vi "24HP test panel - USB - external control.vi"(2 "Datalog file path (full)":path, 3 "COM port":refnum<visa-resource-name>, 4 "Log data stream":bool, 5 "Data rate (Hz)":u8(ring)=14 items=["1", "2", "4", "5", "8", "10", "16", "20", "25", "32", "40", "50", "64", "80", "100", "125", "160", "200", "250", "320", "400", "500", "625", "800", "1000"], 6 "N samples":u32=1000, 7 "Command":T2="D") -> (0 "Error":errorcluster, 1 "Data out":T3[](array[typedef]) {"Time stamp" format="%<%.6X\n%x>T"})   [LabVIEW 2020]
uses:
  ctls/24HP_Cmd (USB).ctl
  ctls/24HP_Data cluster.ctl
  Globals/Meas_global.vi
panel:
  in  "Main":T1(tab)
  out "Serial number":u32
  out "Subsystems ok":bool[](array[boolean])
  out "Pressure sensor values in range":bool[](array[boolean])
  out "Pressure sensor status good":bool[](array[boolean])
  out "P_offset_table_auto_zero":sgl[][](array[numeric]) format="%#_6f"
  out "n":u16
  out "Auto zero progBar":u16(slide) caption="Collecting samples, please maintain dP = 0" scale=0.0..100.0
  in  "P_atm offset (Pa)":sgl
  in  "T_external offset (°C)":sgl
  in  "Data period on power-up (ms)":u32=10000
  in  "TTL baud rate (bps)":u32=500000
  in  "Serial number":u32=9999
  in  "IMU params 2":u8[](array[numeric])=[0, 0, 4]
  in  "IMU params 1":sgl[](array[numeric])=[1.0, 0.0, 0.0, 0.0]
  in  "P_offset_table":sgl[][](array[numeric])=[[0.0, 0.0, 0.0, 0.0, 0.0, 0.0, 0.0, 0.0], [0.0, 0.0, 0.0, 0.0, 0.0, 0.0, 0.0, 0.0], [0.0, 0.0, 0.0, 0.0, 0.0, 0.0, 0.0, 0.0]] format="%#_6f"
  in  "Power-up defaults":u8[](array[numeric])=[0, 3, 0, 0]
  out "Chk ok":bool
  out "EEPROM Checksum":u16 format="%04x"
  out "received":bool
  out "Returned data rate (Hz)":u32
  out "sent":bool
  out "w_xyz (dps)":sgl[](array[numeric])
  out "a_xyz (g)":sgl[](array[numeric])
  out "T_external (°C)":sgl format="%#_4f"
  out "T_board (°C)":sgl format="%#_4f"
  out "Sensor status":bool[][][](array[boolean])
  out "frm err":u32
  out "chk err":u32
  in  "Stop Data":bool
  out "Checksum ok":bool
  out "Stream enabled":bool
  out "Pressures":sgl[][](graph)
  out "Rel. hum (%)":sgl format="%#_4f"
  out "P_atm (mbar)":sgl format="%#_4f"
  # "Paul Nathan"
  # "11/2021"
  # "On-board temperature sensor ok"
  # "External temperature sensor ok"
  # "MCU EEPROM checksum ok"
  # "IMU detected"
  # "Accelerometer self test pass"
  # "Gyroscope self test pass"
  # "Env. sensor detected"
  # "Bank 0 pressure sensor values in range"
  # "Bank 1 pressure sensor values in range"
  # "Bank 2 pressure sensor values in range"
  # "Bank 0 pressure sensor statuses good"
  # "Bank 1 pressure sensor statuses good"
  # "Bank 2 pressure sensor statuses good"
  # "%"
  # "P0 offset"
  # "P1 offset"
  # "P2 offset"
  # "P3 offset"
  # "P4 offset"
  # "P5 offset"
  # "P6 offset"
  # "P7 offset"
  # "Bank 2"
  # "Bank 1"
  # "Bank 0"
  # "acc range mode"
  # "gyr range mode"
  # "IMU update rate mode"
  # "a_xyz scale"
  # "w_x offset (dps)"
  # "w_y offset (dps)"
  # "w_z offset (dps)"
  # "P0 offset"
  # "P1 offset"
  # "P2 offset"
  # "P3 offset"
  # "P4 offset"
  # "P5 offset"
  # "P6 offset"
  # "P7 offset"
  # "Bank 2"
  # "Bank 1"
  # "Bank 0"
  # "TTL data output on power-up"
  # "Number of active sensor banks"
  # "Sleep sensors after data stream"
  # "Sync sensor and data clocks"
  # "bank"
  # "0"
  # "1"
  # "2"
  # "3"
  # "4"
  # "5"
  # "6"
  # "7"
  # "Powered"
  # "!Busy"
  # "!MemErr"
  # "!MathSat"
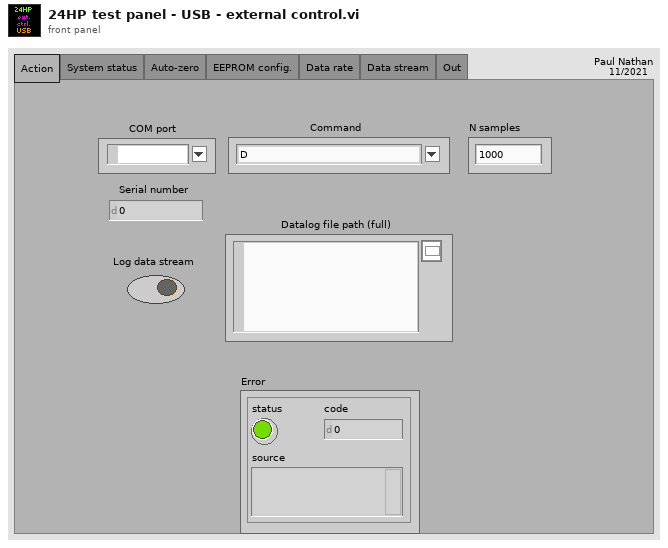
[diagram p1: front panel]
types:
  T1 = enum32{"Action", "System status", "Auto-zero", "EEPROM config.", "Data rate", "Data stream", "Out"}
  T2 = typedef "24HP_Cmd (USB).ctl" = string
  T3 = typedef "24HP_Data cluster.ctl" = cluster{"Time stamp":timestamp, "Pressures (Pa)":sgl[], "T_external (°C)":sgl, "T_board (°C)":sgl, "P_atm (mbar)":sgl, "Rel. hum. (%)":sgl, "a_xyz (g)":sgl[], "w_xyz (dps)":sgl[], "Status bytes":u8[]}
  T4 = enum32{"Action", "System status", "Auto-zero", "EEPROM config.", "Data rate", "Data stream"}
  T5 = enum16{"open", "replace", "create", "open or create", "replace or create", "replace or create with confirmation"}
  T6 = typedef "Rendezvous RefNum" = refnum<k1>
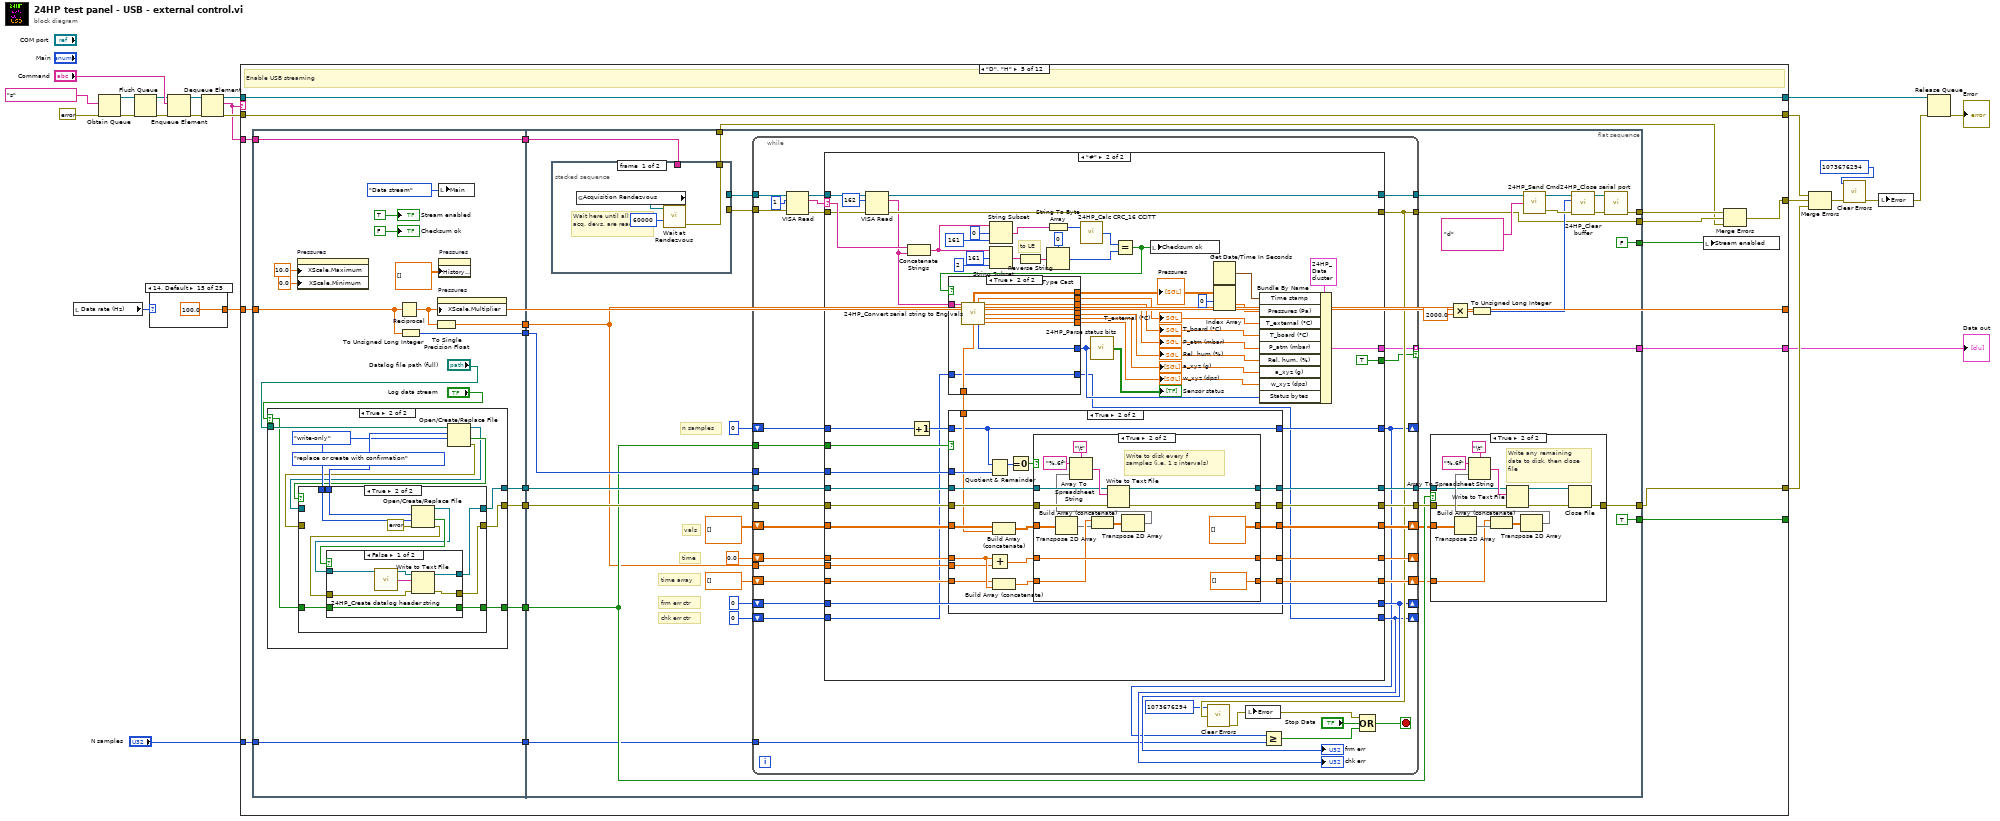
[diagram p0: block diagram]
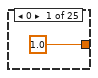
[diagram p2: hidden frame]
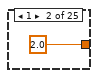
[diagram p3: hidden frame]
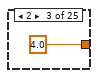
[diagram p4: hidden frame]
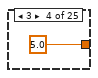
[diagram p5: hidden frame]
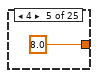
[diagram p6: hidden frame]
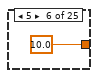
[diagram p7: hidden frame]
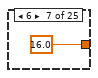
[diagram p8: hidden frame]
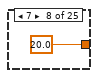
[diagram p9: hidden frame]
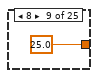
[diagram p10: hidden frame]
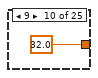
[diagram p11: hidden frame]
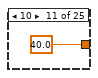
[diagram p12: hidden frame]
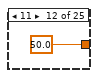
[diagram p13: hidden frame]
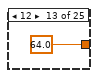
[diagram p14: hidden frame]
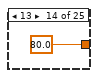
[diagram p15: hidden frame]
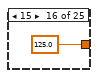
[diagram p16: hidden frame]
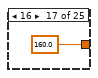
[diagram p17: hidden frame]
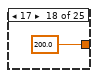
[diagram p18: hidden frame]
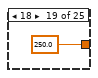
[diagram p19: hidden frame]
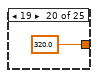
[diagram p20: hidden frame]
diagram:
  n1 = local read "Data rate (Hz)"() -> (w6:u8)
  n2 = Obtain Queue(element data type=T2 "s" ("Combo Box"), error in (no error)=errorcluster {"status"=FALSE, "code"=0, "source"=""}) -> (queue out=w22:refnum<queue>, error out=w23:errorcluster)  [unwired: 3 in, 1 out]
  n3 = Flush Queue(queue=w22, error in (no error)=w23) -> (queue out=w16:refnum<queue>, error out=w15:errorcluster)  [unwired: 1 out]
  n4 = case shown="14, Default" w6 {
    tunnel: [1.0 2.0 4.0 5.0 8.0 10.0 16.0 20.0 25.0 32.0 40.0 50.0 64.0 80.0 100.0 125.0 160.0 200.0 250.0 320.0 400.0 500.0 625.0 800.0 1000.0] -> w5
    frame 0 {
    }
    frame 1 {
    }
    frame 2 {
    }
    frame 3 {
    }
    frame 4 {
    }
    frame 5 {
    }
    frame 6 {
    }
    frame 7 {
    }
    frame 8 {
    }
    frame 9 {
    }
    frame 10 {
    }
    frame 11 {
    }
    frame 12 {
    }
    frame 13 {
    }
    frame 14, Default {
    }
    frame 15 {
    }
    frame 16 {
    }
    frame 17 {
    }
    frame 18 {
    }
    frame 19 {
    }
    frame 20 {
    }
    frame 21 {
    }
    frame 22 {
    }
    frame 23 {
    }
    frame 24 {
    }
  }
  n5 = Enqueue Element(queue=w16, element="Command", error in (no error)=w15) -> (queue out=w20:refnum<queue>, error out=w19:errorcluster)  [unwired: 1 in, 1 out]
  n6 = Dequeue Element(queue=w20, error in (no error)=w19) -> (queue out=w14:refnum<queue>, element=w12:T2, error out=w13:errorcluster)  [unwired: 1 in, 1 out]
  n7 = case shown="\"D\", \"H\"" w12 {
    tunnel: [w56 w93 w144 w269 w378 w664 w691 w753 w795 w824 FALSE FALSE] -> _
    tunnel: w14 -> [w55 w92 w143 w272 w377 w666 w693 w755 w794 w816 w840 w845]
    tunnel: [w55 w92 w143 w272 w377 w666 w693 w755 w794 w815 w840 w845] -> w4
    tunnel: w13 -> [w54 w91 w142 w271 w376 w665 w694 w756 w793 w823 w839 w844]
    tunnel: [w54 w91 w142 w271 w376 w665 w694 w756 w793 w823 w839 w844] -> w11
    tunnel: w12 -> [w53 w90 w141 w277 w375 w668 w698 w761 w792 w822 _ _]
    tunnel: [w51 w88 w139 w270 w363 w667 w692 w754 w790 w817 errorcluster {"status"=FALSE, "code"=0, "source"=""} ("Error out") errorcluster {"status"=FALSE, "code"=0, "source"=""} ("Error out")] -> w10
    tunnel: [_ _ _ _ w373 _ _ _ _ _ _ _] -> w9
    tunnel: w5 -> [w50 w87 w138 w274 w366 w662 _ _ w789 w820 w836 w841]
    tunnel: [w50 w87 w138 w274 w366 w662 w690 w757 w789 w820 w836 w841] -> _
    tunnel: [_ _ _ _ w362 _ _ _ _ _ _ _] -> w2
    tunnel: "N samples" -> [_ _ _ _ w361 _ _ _ _ _ _ _]
    frame "S", "s" {
      # "Perform self-test and retrieve status bytes, Retrieve status bytes"
      n8 = flat-sequence {
        tunnel: w53 -> [w59]
        tunnel: [w59] -> w52
        tunnel: [TRUE] -> w56
        tunnel: w52 -> [w64]
        tunnel: [w63] -> w51
        frame #0 {
          w58 = bool[] [] ("Pressure sensor EEPROM checksums ok")
          n9 = local write "Main"(T4."System status" ("Main")) -> ()
          "Pressure sensor status good" <- w58
          "Pressure sensor values in range" <- w58
          "Subsystems ok" <- w58
        }
        frame #1 {
          w68 = 1 ("length (rest)")
          w75 = u8 0 ("byte count")
          n10 = local read "COM port"() -> (w65:refnum<visa-resource-name>)
          n11 = call "24HP_Open serial port.vi"("timeout (ms)"=u32 5000, "VISA resource name"=w65) -> ("Error out"=w84:errorcluster, "VISA resource name out"=w85:refnum<visa-resource-name>)  [unwired: 8 in]
          n12 = call "24HP_Send Cmd.vi"("Error In"=w84, "Operation"=w64, "Port"=w85) -> ("Error Out"=w82:errorcluster, "Port out"=w83:refnum<visa-resource-name>)  [unwired: 1 in]
          n13 = VISA Read(VISA resource name=w83, byte count=u32 3, error in (no error)=w82) -> (VISA resource name out=w80:refnum<visa-resource-name>, read buffer=w71:string, error out=w79:errorcluster)  [unwired: 1 out]
          n14 = call "24HP_Close serial port.vi"("Error in"=w79, "VISA resource name"=w80) -> ("Error out"=w63:errorcluster)  [unwired: 9 in]
          n15 = String Subset(string=w71, offset (0)=0, length (rest)=w68) -> (substring=w78:string)
          n16 = String Subset(string=w71, offset (0)=1, length (rest)=w68) -> (substring=w77:string)
          n17 = String Subset(string=w71, offset (0)=2 ("length (rest)"), length (rest)=w68) -> (substring=w76:string)
          n18 = Type Cast(type=w75, x=w78) -> (*(type *) &x=w74:u8)
          n19 = Type Cast(type=w75, x=w77) -> (*(type *) &x=w73:u8)
          n20 = Type Cast(type=w75, x=w76) -> (*(type *) &x=w72:u8)
          n21 = Number To Boolean Array(number=w74) -> (Boolean array=w62:bool[])
          n22 = Number To Boolean Array(number=w73) -> (Boolean array=w61:bool[])
          n23 = Number To Boolean Array(number=w72) -> (Boolean array=w60:bool[])
          n24 = local write "Pressure sensor values in range"(w62) -> ()
          n25 = local write "Pressure sensor status good"(w61) -> ()
          n26 = local write "Subsystems ok"(w60) -> ()
        }
      }
    }
    frame "Z", "z" {
      # "Perform permanent auto-zero (write values to EEPROM), Perform temporary auto-zero"
      n27 = flat-sequence {
        tunnel: w90 -> [w97]
        tunnel: [w97] -> w89
        tunnel: [TRUE] -> w93
        tunnel: w89 -> [w109]
        tunnel: [w106] -> w88
        frame #0 {
          n28 = local write "Main"(T4."Auto-zero" ("Main")) -> ()
          "P_offset_table_auto_zero" <- sgl[][] [] ("P_raw_Azero")
          "Auto zero progBar" <- u16 0 ("Collecting samples, please maintain dP = 0")
        }
        frame #1 {
          w98 = 3  # N banks
          # "Reverse columns to match physical layout"
          n29 = local read "COM port"() -> (w110:refnum<visa-resource-name>)
          n30 = call "24HP_Open serial port.vi"("timeout (ms)"=u32 16000, "VISA resource name"=w110) -> ("Error out"=w117:errorcluster, "VISA resource name out"=w118:refnum<visa-resource-name>)  [unwired: 8 in]
          n31 = call "24HP_Send Cmd.vi"("Error In"=w117, "Operation"=w109, "Port"=w118) -> ("Error Out"=w115:errorcluster, "Port out"=w116:refnum<visa-resource-name>)  [unwired: 1 in]
          n32 = VISA Read(VISA resource name=w116, byte count=u32 96, error in (no error)=w115) -> (VISA resource name out=w113:refnum<visa-resource-name>, read buffer=w107:string, error out=w112:errorcluster)  [unwired: 1 out]
          n33 = for {
            N: 100 -> [_]
            shift-right: [w127] -> _
            shift-left: u16 0 -> [w128]
            n34 = Increment(x=w128) -> (x+1=w127:u16)
            "n" <- w127
            n35 = Wait (ms)(milliseconds to wait=u32 100) -> ()  [unwired: 1 out]
            n36 = local write "Auto zero progBar"(w127) -> ()
          }
          n37 = for {
            N: 24 -> [_]
            tunnel: [w131] -> w99 mode=indexing
            tunnel: w107 -> [w130]
            i -> [w137]
            w135 = 4 ("x")
            # "to BE"
            n38 = Multiply(x=w135, y=w137) -> (x*y=w136:i32)
            n39 = String Subset(string=w130, offset (0)=w136, length (rest)=w135) -> (substring=w134:string)
            n40 = Reverse String(1:w134) -> (0:w133:string)
            n41 = Type Cast(type=sgl 0.0 ("byte count"), x=w133) -> (*(type *) &x=w131:sgl)
          }
          n42 = call "24HP_Close serial port.vi"("Error in"=w112, "VISA resource name"=w113) -> ("Error out"=w106:errorcluster)  [unwired: 9 in]
          n43 = for {
            N: w98 -> [_]
            tunnel: w99 -> [w124]
            tunnel: [w121] -> w100 mode=indexing
            i -> [w123]
            w120 = 8 ("x")
            n44 = Multiply(x=w120, y=w123) -> (x*y=w122:i32)
            n45 = Array Subset(array=w124, index=w122, length=w120) -> (w121:sgl[])
          }
          n46 = Transpose 2D Array(2D array=w100) -> (transposed array=w103:sgl[][])
          n47 = for {
            tunnel: w103 -> [w126] mode=indexing
            tunnel: [w125] -> w101 mode=indexing
            n48 = Reverse 1D Array(array=w126) -> (reversed array=w125:sgl[])
          }
          n49 = Transpose 2D Array(2D array=w101) -> (transposed array=w102:sgl[][])
          n50 = local write "P_offset_table_auto_zero"(w102) -> ()
        }
      }
    }
    frame "e" {
      # "Read all EEPROM values"
      n51 = flat-sequence {
        tunnel: w141 -> [w157]
        tunnel: [w157] -> w140
        tunnel: [TRUE] -> w144
        tunnel: w140 -> [w225]
        tunnel: [w223] -> w139
        frame #0 {
          n52 = local write "Data period on power-up (ms)"(u32 0 ("Data period on power-up (ms)")) -> ()
          n53 = local write "T_external offset (°C)"(sgl 0.0 ("T_external offset (°C)")) -> ()
          n54 = local write "EEPROM Checksum"(u16 0 ("EEPROM Checksum")) -> ()
          n55 = local write "TTL baud rate (bps)"(u32 0 ("TTL baud rate (bps)")) -> ()
          n56 = local write "Main"(T4."EEPROM config." ("Main")) -> ()
          n57 = local write "Power-up defaults"(u8[] [] ("Power-up defaults")) -> ()
          n58 = local write "P_atm offset (Pa)"(sgl 0.0 ("P_atm offset (Pa)")) -> ()
          n59 = local write "P_offset_table"(sgl[][] [] ("EEPROM array")) -> ()
          n60 = local write "Serial number"(u32 0 ("Serial number")) -> ()
          n61 = local write "IMU params 1"(sgl[] []) -> ()
          n62 = local write "IMU params 2"(u8[] []) -> ()
          n63 = local write "Chk ok"(FALSE ("Chk ok")) -> ()
        }
        frame #1 {
          w165 = 3  # N banks
          w197 = u32 2 ("y")
          w199 = u32 141 ("byte count")
          # "to BE"
          # "Reverse columns to match physical layout"
          # "to BE"
          n64 = local read "COM port"() -> (w226:refnum<visa-resource-name>)
          n65 = call "24HP_Open serial port.vi"("timeout (ms)"=u32 5000, "VISA resource name"=w226) -> ("Error out"=w232:errorcluster, "VISA resource name out"=w233:refnum<visa-resource-name>)  [unwired: 8 in]
          n66 = call "24HP_Send Cmd.vi"("Error In"=w232, "Operation"=w225, "Port"=w233) -> ("Error Out"=w230:errorcluster, "Port out"=w231:refnum<visa-resource-name>)  [unwired: 1 in]
          n67 = VISA Read(VISA resource name=w231, byte count=w199, error in (no error)=w230) -> (VISA resource name out=w229:refnum<visa-resource-name>, read buffer=w159:string, error out=w228:errorcluster)  [unwired: 1 out]
          n68 = Subtract(x=w199, y=w197) -> (x-y=w198:u32)
          n69 = call "24HP_Close serial port.vi"("Error in"=w228, "VISA resource name"=w229) -> ("Error out"=w223:errorcluster)  [unwired: 9 in]
          n70 = String Subset(string=w159, offset (0)=0, length (rest)=96 ("length (rest)")) -> (substring=w222:string)
          n71 = String Subset(string=w159, offset (0)=96, length (rest)=4 ("length (rest)")) -> (substring=w196:string)
          n72 = String Subset(string=w159, offset (0)=100, length (rest)=4 ("length (rest)")) -> (substring=w160:string)
          n73 = String Subset(string=w159, offset (0)=104, length (rest)=4 ("length (rest)")) -> (substring=w215:string)
          n74 = String Subset(string=w159, offset (0)=108, length (rest)=4 ("length (rest)")) -> (substring=w205:string)
          n75 = String Subset(string=w159, offset (0)=112, length (rest)=4 ("length (rest)")) -> (substring=w191:string)
          n76 = String Subset(string=w159, offset (0)=116, length (rest)=4 ("length (rest)")) -> (substring=w180:string)
          n77 = String Subset(string=w159, offset (0)=120, length (rest)=16 ("length (rest)")) -> (substring=w174:string)
          n78 = String Subset(string=w159, offset (0)=136, length (rest)=3 ("length (rest)")) -> (substring=w170:string)
          n79 = String Subset(string=w159, offset (0)=w198, length (rest)=w197) -> (substring=w209:string)
          n80 = String Subset(string=w159, offset (0)=0, length (rest)=w198) -> (substring=w207:string)
          n81 = for {
            N: 24 -> [_]
            tunnel: [w253] -> w166 mode=indexing
            tunnel: w222 -> [w252]
            i -> [w257]
            w255 = 4 ("x")
            # "to BE"
            n82 = Multiply(x=w255, y=w257) -> (x*y=w256:i32)
            n83 = String Subset(string=w252, offset (0)=w256, length (rest)=w255) -> (substring=w251:string)
            n84 = Reverse String(1:w251) -> (0:w250:string)
            n85 = Type Cast(type=sgl 0.0 ("byte count"), x=w250) -> (*(type *) &x=w253:sgl)
          }
          n86 = for {
            N: 4 -> [_]
            tunnel: [w243] -> w173 mode=indexing
            tunnel: w174 -> [w242]
            i -> [w247]
            w245 = 4 ("x")
            # "to BE"
            n87 = Multiply(x=w245, y=w247) -> (x*y=w246:i32)
            n88 = String Subset(string=w242, offset (0)=w246, length (rest)=w245) -> (substring=w241:string)
            n89 = Reverse String(1:w241) -> (0:w240:string)
            n90 = Type Cast(type=sgl 0.0 ("byte count"), x=w240) -> (*(type *) &x=w243:sgl)
          }
          n91 = Reverse String(1:w196) -> (0:w192:string)
          n92 = Reverse String(1:w160) -> (0:w164:string)
          n93 = Reverse String(1:w215) -> (0:w219:string)
          n94 = Reverse String(1:w205) -> (0:w201:string)
          n95 = Reverse String(1:w191) -> (0:w187:string)
          n96 = String To Byte Array(string=w180) -> (unsigned byte array=w181:u8[])
          n97 = String To Byte Array(string=w170) -> (unsigned byte array=w169:u8[])
          n98 = Reverse String(1:w209) -> (0:w211:string)
          n99 = String To Byte Array(string=w207) -> (unsigned byte array=w214:u8[])
          n100 = call "24HP_Calc CRC_16 CCITT.vi"("Data bytes"=w214) -> ("CRC_16-CCITT"=w213:u16)  [unwired: 1 in]
          n101 = Type Cast(type=sgl 0.0 ("byte count"), x=w192) -> (*(type *) &x=w182:sgl)
          n102 = Type Cast(type=sgl 0.0 ("byte count"), x=w164) -> (*(type *) &x=w158:sgl)
          n103 = Type Cast(type=u32 0 ("byte count"), x=w219) -> (*(type *) &x=w200:u32)
          n104 = Type Cast(type=u32 0 ("byte count"), x=w201) -> (*(type *) &x=w183:u32)
          n105 = Type Cast(type=u32 0 ("byte count"), x=w187) -> (*(type *) &x=w184:u32)
          n106 = Type Cast(type=u16 0 ("byte count"), x=w211) -> (*(type *) &x=w206:u16)
          n107 = Equal?(x=w206, y=w213) -> (x = y?=w212:bool)
          n108 = for {
            N: w165 -> [_]
            tunnel: w166 -> [w239]
            tunnel: [w236] -> w167 mode=indexing
            i -> [w238]
            w235 = 8 ("x")
            n109 = Multiply(x=w235, y=w238) -> (x*y=w237:i32)
            n110 = Array Subset(array=w239, index=w237, length=w235) -> (w236:sgl[])
          }
          n111 = Transpose 2D Array(2D array=w167) -> (transposed array=w179:sgl[][])
          n112 = for {
            tunnel: w179 -> [w249] mode=indexing
            tunnel: [w248] -> w178 mode=indexing
            n113 = Reverse 1D Array(array=w249) -> (reversed array=w248:sgl[])
          }
          n114 = Transpose 2D Array(2D array=w178) -> (transposed array=w177:sgl[][])
          n115 = local write "P_offset_table"(w177) -> ()
          n116 = local write "T_external offset (°C)"(w182) -> ()
          n117 = local write "P_atm offset (Pa)"(w158) -> ()
          n118 = local write "Serial number"(w200) -> ()
          n119 = local write "Data period on power-up (ms)"(w183) -> ()
          n120 = local write "TTL baud rate (bps)"(w184) -> ()
          n121 = local write "Power-up defaults"(w181) -> ()
          n122 = local write "IMU params 1"(w173) -> ()
          n123 = local write "IMU params 2"(w169) -> ()
          n124 = local write "EEPROM Checksum"(w206) -> ()
          n125 = local write "Chk ok"(w212) -> ()
        }
      }
    }
    frame "E" {
      # "Write all EEPROM values (including new checksum)"
      n126 = flat-sequence {
        tunnel: w277 -> [w298]
        tunnel: [w298] -> w276
        tunnel: [w289] -> w275
        tunnel: ["Data period on power-up (ms)"] -> w273
        tunnel: ["Serial number"] -> w268
        tunnel: ["TTL baud rate (bps)"] -> w265
        tunnel: ["T_external offset (°C)"] -> w264
        tunnel: ["IMU params 1"] -> w263
        tunnel: ["IMU params 2"] -> w262
        tunnel: ["Power-up defaults"] -> w259
        tunnel: ["P_atm offset (Pa)"] -> w258
        tunnel: [TRUE] -> w269
        tunnel: w276 -> [w338]
        tunnel: w275 -> [w336]
        tunnel: [w335] -> w270
        tunnel: w273 -> [w328]
        tunnel: w268 -> [w322]
        tunnel: w265 -> [w320]
        tunnel: w264 -> [w316]
        tunnel: w263 -> [w311]
        tunnel: w262 -> [w313]
        tunnel: [w308] -> w261
        tunnel: [TRUE ("Chk ok")] -> w260
        tunnel: w259 -> [w306]
        tunnel: w258 -> [w303]
        frame #0 {
          # "Reverse columns back to logical layout"
          n127 = local write "Main"(T4."EEPROM config." ("Main")) -> ()
          n128 = local write "Chk ok"(FALSE ("Chk ok")) -> ()
          n129 = Transpose 2D Array(2D array="P_offset_table") -> (transposed array=w292:sgl[][])
          n130 = for {
            tunnel: w292 -> [w300] mode=indexing
            tunnel: [w299] -> w291 mode=indexing
            n131 = Reverse 1D Array(array=w300) -> (reversed array=w299:sgl[])
          }
          n132 = Transpose 2D Array(2D array=w291) -> (transposed array=w289:sgl[][])
        }
        frame #1 {
          w301 = ""
          # "to LE"
          n133 = local read "COM port"() -> (w339:refnum<visa-resource-name>)
          n134 = for {
            tunnel: w336 -> [w352] mode=indexing
            shift-right: [w351] -> w331
            shift-left: "" -> [w350]
            n135 = for {
              tunnel: w352 -> [w355] mode=indexing
              shift-right: [w356] -> w351
              shift-left: w350 -> [w357]
              # "to LE"
              n136 = Type Cast(type="", x=w355) -> (*(type *) &x=w354:string)
              n137 = Reverse String(1:w354) -> (0:w353:string)
              n138 = Concatenate Strings(w357, w353) -> (w356:string)
            }
          }
          n139 = for {
            tunnel: w311 -> [w346] mode=indexing
            shift-right: [w347] -> w309
            shift-left: "" -> [w348]
            # "to LE"
            n140 = Type Cast(type="", x=w346) -> (*(type *) &x=w345:string)
            n141 = Reverse String(1:w345) -> (0:w344:string)
            n142 = Concatenate Strings(w348, w344) -> (w347:string)
          }
          n143 = Type Cast(type=w301, x=w316) -> (*(type *) &x=w317:string)
          n144 = Type Cast(type=w301, x=w303) -> (*(type *) &x=w304:string)
          n145 = Type Cast(type=w301, x=w322) -> (*(type *) &x=w323:string)
          n146 = Type Cast(type=w301, x=w328) -> (*(type *) &x=w329:string)
          n147 = Type Cast(type=w301, x=w320) -> (*(type *) &x=w319:string)
          n148 = Type Cast(type=w301, x=w313) -> (*(type *) &x=w312:string)
          n149 = Reverse String(1:w317) -> (0:w315:string)
          n150 = Reverse String(1:w304) -> (0:w302:string)
          n151 = Reverse String(1:w323) -> (0:w321:string)
          n152 = Reverse String(1:w329) -> (0:w324:string)
          n153 = Reverse String(1:w319) -> (0:w318:string)
          n154 = Byte Array To String(unsigned byte array=w306) -> (string=w305:string)
          n155 = call "24HP_Open serial port.vi"("timeout (ms)"=u32 5000, "VISA resource name"=w339) -> ("Error out"=w341:errorcluster, "VISA resource name out"=w342:refnum<visa-resource-name>)  [unwired: 8 in]
          n156 = Concatenate Strings(w331, w315, w302, w321, w324, w318, w305, w309, w312) -> (w330:string)
          n157 = String To Byte Array(string=w330) -> (unsigned byte array=w327:u8[])
          n158 = call "24HP_Calc CRC_16 CCITT.vi"("Data bytes"=w327) -> ("CRC_16-CCITT"=w308:u16)  [unwired: 1 in]
          n159 = Type Cast(type="", x=w308) -> (*(type *) &x=w326:string)
          n160 = Reverse String(1:w326) -> (0:w325:string)
          n161 = Concatenate Strings(w330, w325) -> (w334:string)
          n162 = call "24HP_Send Cmd + Data.vi"("Error In"=w341, "Data"=w334, "Operation"=w338, "Port"=w342) -> ("Error Out"=w332:errorcluster, "Port out"=w333:refnum<visa-resource-name>)  [unwired: 1 in]
          n163 = call "24HP_Close serial port.vi"("Error in"=w332, "VISA resource name"=w333) -> ("Error out"=w335:errorcluster)  [unwired: 9 in]
        }
      }
      n164 = flat-sequence {
        tunnel: [w278] -> w267
        tunnel: w269 -> [w278]
        tunnel: [w280] -> w266
        tunnel: w267 -> [w280]
        tunnel: [w282] -> _
        tunnel: w266 -> [w282]
        frame #0 {
          n165 = local write "Main"(T4."Action" ("Main")) -> ()
        }
        frame #1 {
          n166 = One Button Dialog(message="Application restart required after making changes to the EEPROM.\nThe application will now exit. Please re-run.") -> ()  [unwired: 1 in, 1 out]
        }
        frame #2 {
          n167 = Stop(stop? (T)=TRUE) -> ()
        }
      }
      "EEPROM Checksum" <- w261
      "Chk ok" <- w260
    }
    frame "D", "H" {
      # "Enable USB streaming"
      n168 = flat-sequence {
        tunnel: w375 -> [w395]
        tunnel: [w395] -> w374
        tunnel: [w392] -> w372
        tunnel: [w391] -> w371
        tunnel: [w390] -> w370
        tunnel: w366 -> [w382]
        tunnel: [w388] -> w369
        tunnel: [w384] -> w368
        tunnel: w361 -> [w379]
        tunnel: [w379] -> w360
        tunnel: [TRUE] -> w378
        tunnel: w374 -> [w437]
        tunnel: [w467] -> w364
        tunnel: [w466] -> w373
        tunnel: w372 -> [w463]
        tunnel: w371 -> [w462]
        tunnel: w370 -> [w464]
        tunnel: w369 -> [w446]
        tunnel: w368 -> [w456]
        tunnel: [FALSE] -> w367
        tunnel: [w440] -> w365
        tunnel: [w436] -> w362
        tunnel: w360 -> [w435]
        tunnel: [w434] -> w359
        frame #0 {
          n169 = case shown="True" "Log data stream" {
            selector: "Log data stream" -> [w396 w399]
            tunnel: "Datalog file path (full)" -> [_ w408]
            tunnel: [refnum<file> refnum ("refnum out") w405] -> w392
            tunnel: [errorcluster {"status"=FALSE, "code"=0, "source"=""} ("error out") w404] -> w391
            tunnel: [w396 w400] -> w384
            frame False {
            }
            frame True {
              w406 = enum16{"read/write", "read-only", "write-only"}."write-only" ("access (0:read/write)")
              w407 = T5."replace or create with confirmation" ("operation (0:open)")
              n170 = Open/Create/Replace File(file path (use dialog)=w408, operation (0:open)=w407, access (0:read/write)=w406) -> (refnum out=w401:refnum<file>, cancelled=w403:bool, error out=w402:errorcluster)  [unwired: 3 in]
              n171 = case shown="True" w403 {
                tunnel: w407 -> [_ w424]
                tunnel: w406 -> [_ w423]
                tunnel: w402 -> [w412 _]
                tunnel: [w410 w418] -> w405
                tunnel: [w411 w419] -> w404
                tunnel: w401 -> [w413 _]
                tunnel: [w409 w416] -> w400
                tunnel: w399 -> [w409 w415]
                frame False {
                  n172 = call "24HP_Create datalog header string.vi"() -> ("Datalog header string"=w414:string)  [unwired: 1 in]
                  n173 = Write to Text File(file (use dialog)=w413, text=w414, error in=w412) -> (refnum out=w410:refnum<file>, error out=w411:errorcluster)  [unwired: 1 in, 1 out]
                }
                frame True {
                  n174 = Open/Create/Replace File(error in=errorcluster {"status"=FALSE, "code"=0, "source"=""}, operation (0:open)=w424, access (0:read/write)=w423) -> (refnum out=w421:refnum<file>, cancelled=w422:bool, error out=w420:errorcluster)  [unwired: 3 in]
                  n175 = case shown="False" w422 {
                    tunnel: w421 -> [w429 _]
                    tunnel: w420 -> [w428 _]
                    tunnel: [w427 errorcluster {"status"=FALSE, "code"=0, "source"=""} ("error out")] -> w419
                    tunnel: [w426 refnum<file> refnum ("t")] -> w418
                    tunnel: [w425 w431] -> w416
                    tunnel: w415 -> [w425 _]
                    frame False {
                      n176 = call "24HP_Create datalog header string.vi"() -> ("Datalog header string"=w430:string)  [unwired: 1 in]
                      n177 = Write to Text File(file (use dialog)=w429, text=w430, error in=w428) -> (refnum out=w426:refnum<file>, error out=w427:errorcluster)  [unwired: 1 in, 1 out]
                    }
                    frame True {
                      w431 = FALSE ("Log data stream")
                      n178 = local write "Log data stream"(w431) -> ()
                    }
                  }
                }
              }
            }
          }
          n179 = property on="Pressures" class="WFChart (strict)"("XScale.Maximum"=10.0 ("X Scale.Range:Maximum"), "XScale.Minimum"=0.0 ("X Scale.Range:Minimum")) -> ()  [unwired: 2 in, 2 out]
          n180 = Reciprocal(x=w382) -> (1/x=w389:dbl)
          n181 = To Unsigned Long Integer(number=w382) -> (unsigned 32bit integer=w390:u32)
          n182 = To Single Precision Float(number=w389) -> (single precision float=w388:sgl)
          n183 = property on="Pressures" class="WFChart (strict)"("XScale.Multiplier"=w389) -> ()  [unwired: 2 in, 2 out]
          n184 = local write "Main"(T4."Data stream" ("Main")) -> ()
          n185 = property on="Pressures" class="WFChart (strict)"("History Data"=sgl[][] []) -> ()  [unwired: 2 in, 2 out]
          "Checksum ok" <- FALSE ("Checksum ok")
          "Stream enabled" <- TRUE ("Stream enabled")
        }
        frame #1 {
          # "n samples"
          # "chk err ctr"
          # "frm err ctr"
          # "vals"
          # "time"
          # "time array"
          n186 = stacked-sequence {
            tunnel: [_ w476] -> w455
            tunnel: [_ w474] -> w454
            tunnel: w437 -> [_ w473]
            tunnel: [w469 _] -> w434
            frame #0 {
              # "Wait here until all acq. devs. are ready."
              n187 = global read "Meas_global.vi" "Acquisition Rendezvous"() -> (w470:T6)
              n188 = call <vilib>:"Wait at Rendezvous.vi"("ms timeout (-1)"=60000, "rendezvous"=w470) -> ("error out"=w469:errorcluster)  [unwired: 3 in, 2 out]
            }
            frame #1 {
              n189 = case shown="\"H\"" w473 {
                tunnel: [u32 15000 ("timeout (ms)") u32 5000 ("timeout (ms)")] -> w472
                frame "H" {
                }
                frame "D", Default {
                }
              }
              n190 = local read "COM port"() -> (w478:refnum<visa-resource-name>)
              n191 = call "24HP_Open serial port.vi"("timeout (ms)"=w472, "VISA resource name"=w478) -> ("Error out"=w475:errorcluster, "VISA resource name out"=w477:refnum<visa-resource-name>)  [unwired: 8 in]
              n192 = call "24HP_Send Cmd.vi"("Error In"=w475, "Operation"=w473, "Port"=w477) -> ("Error Out"=w474:errorcluster, "Port out"=w476:refnum<visa-resource-name>)  [unwired: 1 in]
            }
          }
          n193 = while {
            tunnel: [w492] -> w440
            tunnel: w455 -> [w494]
            tunnel: [w511] -> w453
            shift-right: [w482] -> _
            shift-left: u32 0 -> [w508]
            tunnel: w464 -> [w507]
            tunnel: w463 -> [w506]
            tunnel: w462 -> [w505]
            tunnel: [w504] -> w461
            tunnel: [w503] -> w460
            shift-right: [w502] -> w443
            shift-left: sgl[][] [] -> [w501]
            shift-right: [w498] -> _
            shift-left: sgl 0.0 ("Numeric") -> [w500]
            tunnel: w446 -> [w499]
            shift-right: [w496] -> w442
            shift-left: sgl[] [] -> [w497]
            tunnel: w456 -> [w495]
            tunnel: w454 -> [w493]
            shift-right: [w487] -> _
            shift-left: u32 0 -> [w489]
            shift-right: [w486] -> _
            shift-left: u32 0 -> [w488]
            tunnel: [w485] -> w436 mode=indexing if=w484
            tunnel: w435 -> [w481]
            stop <- w509 stop-if-true
            n194 = VISA Read(VISA resource name=w494, byte count=u32 1, error in (no error)=w493) -> (VISA resource name out=w513:refnum<visa-resource-name>, read buffer=w514:string, error out=w512:errorcluster)  [unwired: 1 out]
            n195 = case shown="\"#\"" w514 {
              selector: w514 -> [_ w565]
              tunnel: w513 -> [w526 w551]
              tunnel: [w527 w581] -> w492
              tunnel: w512 -> [w527 w550]
              tunnel: [w526 w582] -> w511
              tunnel: w508 -> [w525 w537]
              tunnel: [w525 w580] -> w482
              tunnel: w507 -> [_ w579]
              tunnel: w506 -> [w524 w578]
              tunnel: w505 -> [w523 w577]
              tunnel: [w523 w576] -> w504
              tunnel: [w524 w575] -> w503
              tunnel: [w522 w574] -> w502
              tunnel: w501 -> [w522 w573]
              tunnel: w500 -> [w521 w572]
              tunnel: w499 -> [_ w571]
              tunnel: [w521 w570] -> w498
              tunnel: w497 -> [w520 w569]
              tunnel: [w520 w568] -> w496
              tunnel: w495 -> [_ w567]
              tunnel: w489 -> [w519 w566]
              tunnel: w488 -> [w518 w535]
              tunnel: [w517 w566] -> w487
              tunnel: [w518 w534] -> w486
              tunnel: [_ w533] -> w485
              tunnel: [FALSE ("Stream enabled") TRUE ("Stream enabled")] -> w484
              frame Default {
                # "Frame error"
                n196 = Increment(x=w519) -> (x+1=w517:u32)
              }
              frame "#" {
                # "to LE"
                n197 = VISA Read(VISA resource name=w551, byte count=u32 162, error in (no error)=w550) -> (VISA resource name out=w582:refnum<visa-resource-name>, read buffer=w549:string, error out=w581:errorcluster)  [unwired: 1 out]
                n198 = Concatenate Strings(w565, w549) -> (w553:string)
                n199 = Increment(x=w537) -> (x+1=w536:u32)
                n200 = String Subset(string=w553, offset (0)=0, length (rest)=161 ("length (rest)")) -> (substring=w552:string)
                n201 = String Subset(string=w553, offset (0)=161, length (rest)=2 ("length (rest)")) -> (substring=w559:string)
                n202 = Reverse String(1:w559) -> (0:w558:string)
                n203 = String To Byte Array(string=w552) -> (unsigned byte array=w563:u8[])
                n204 = Type Cast(type=u16 0 ("length (rest)"), x=w558) -> (*(type *) &x=w557:u16)
                n205 = call "24HP_Calc CRC_16 CCITT.vi"("Data bytes"=w563) -> ("CRC_16-CCITT"=w556:u16)  [unwired: 1 in]
                n206 = Equal?(x=w556, y=w557) -> (x = y?=w547:bool)
                n207 = case shown="True" w547 {
                  tunnel: w549 -> [_ w602]
                  tunnel: [w590 w601] -> w548
                  tunnel: [w591 w594] -> w546
                  tunnel: [w584 w600] -> w538
                  tunnel: [w585 w599] -> w529
                  tunnel: [w585 w598] -> w528
                  tunnel: [w588 w597] -> w539
                  tunnel: [w588 w596] -> w540
                  tunnel: [w586 w595] -> w534
                  tunnel: w535 -> [w587 w595]
                  tunnel: [w585 w593] -> w531
                  tunnel: [w585 w592] -> w530
                  frame False {
                    w584 = u8[] [0, 0, 0, 0, 0, 0, 0, 0, 0, 0, 0, 0, 0, 0, 0, 0, 0, 0, 0, 0, 0, 0, 0, 0] ("All vals")
                    w583 = sgl[] [nan, nan, nan, nan, nan, nan, nan, nan, nan, nan, nan, nan, nan, nan, nan, nan, nan, nan, nan, nan, nan, nan, nan, nan] ("All vals")
                    w588 = sgl[] [nan, nan, nan] ("All vals")
                    w585 = sgl nan ("Numeric")
                    n208 = To Single Precision Float(number=w584) -> (single precision float=w589:sgl[])
                    n209 = Increment(x=w587) -> (x+1=w586:u32)
                    n210 = Build Array(w583) -> (w591:sgl[][])
                    n211 = Build Array (concatenate)(w583, w585, w589) -> (w590:sgl[])
                  }
                  frame True {
                    n212 = call "24HP_Convert serial string to Eng vals.vi"("Serial buffer string (excluding FrameChar)"=w602) -> ("Pressures"=w594:sgl[][], "T_external (°C)"=w593:sgl, "T_board (°C)"=w592:sgl, "P_atmos (mbar)"=w599:sgl, "RH (%)"=w598:sgl, "a_xyz (g)"=w597:sgl[], "All vals"=w601:sgl[], "Status bytes"=w600:u8[], "w_xyz (deg/s)"=w596:sgl[])  [unwired: 6 in]
                  }
                }
                "Pressures" <- w546
                "T_board (°C)" <- w530
                "T_external (°C)" <- w531
                "w_xyz (dps)" <- w540
                "a_xyz (g)" <- w539
                "P_atm (mbar)" <- w529
                "Rel. hum (%)" <- w528
                n213 = case shown="True" w567 {
                  tunnel: w536 -> [w608 w609]
                  tunnel: [w608 w609] -> w580
                  tunnel: w579 -> [_ w627]
                  tunnel: w548 -> [_ w613]
                  tunnel: w578 -> [w606 w624]
                  tunnel: w577 -> [w607 w623]
                  tunnel: [w607 w622] -> w576
                  tunnel: [w606 w621] -> w575
                  tunnel: w573 -> [w605 w614]
                  tunnel: [w605 w620] -> w574
                  tunnel: w572 -> [w604 w617]
                  tunnel: w571 -> [_ w616]
                  tunnel: [w604 w619] -> w570
                  tunnel: w569 -> [w603 w615]
                  tunnel: [w603 w618] -> w568
                  frame False {
                  }
                  frame True {
                    n214 = Add(x=w617, y=w616) -> (x+y=w612:sgl)
                    n215 = Quotient & Remainder(x=w609, y=w627) -> (x-y*floor(x/y)=w626:u32)  [unwired: 1 out]
                    n216 = Build Array (concatenate)(w614, w613) -> (w610:sgl[][])
                    n217 = Build Array (concatenate)(w615, w617) -> (w611:sgl[])
                    n218 = Equal To 0?(x=w626) -> (x = 0?=w625:bool)
                    n219 = case shown="True" w625 {
                      tunnel: w624 -> [w631 w644]
                      tunnel: w623 -> [w632 w643]
                      tunnel: [w632 w642] -> w622
                      tunnel: [w631 w641] -> w621
                      tunnel: w610 -> [w629 w636]
                      tunnel: [w629 sgl[][] []] -> w620
                      tunnel: w612 -> [w630 w639]
                      tunnel: [w630 w639] -> w619
                      tunnel: w611 -> [w628 w638]
                      tunnel: [w628 sgl[] []] -> w618
                      frame False {
                      }
                      frame True {
                        # "Write to disk every f samples (i.e. 1 s intervals)"
                        n220 = Transpose 2D Array(2D array=w636) -> (transposed array=w635:sgl[][])
                        n221 = Build Array (concatenate)(w638, w635) -> (w634:sgl[][])
                        n222 = Transpose 2D Array(2D array=w634) -> (transposed array=w633:sgl[][])
                        n223 = Array To Spreadsheet String(delimiter (Tab)="\t", array=w633, 3:"%.6f" ("format string")) -> (spreadsheet string=w647:string)
                        n224 = Write to Text File(file (use dialog)=w644, text=w647, error in=w643) -> (refnum out=w641:refnum<file>, error out=w642:errorcluster)  [unwired: 1 in, 1 out]
                      }
                    }
                  }
                }
                n225 = call "24HP_Parse status bits.vi"("Status bytes"=w538) -> ("Sensor status"=→"Sensor status":bool[][][])
                n226 = local write "Checksum ok"(w547) -> ()
                n227 = Get Date/Time In Seconds() -> (seconds since 1Jan1904=w543:timestamp)
                n228 = Index Array(array=w546, index (row)=0) -> (element=w542:sgl[])  [unwired: 1 in]
                n229 = Bundle By Name(cluster=T3 {"Time stamp"=timestamp(0 s since 1904-01-01), "Pressures (Pa)"=[], "T_external (°C)"=0.0, "T_board (°C)"=0.0, "P_atm (mbar)"=0.0, "Rel. hum. (%)"=0.0, "a_xyz (g)"=[0.0, 0.0, 0.0], "w_xyz (dps)"=[0.0, 0.0, 0.0], "Status bytes"=[]} ("Data cluster muScan-64"), "Time stamp"=w543, "Pressures (Pa)"=w542, "T_external (°C)"=w531, "T_board (°C)"=w530, "P_atm (mbar)"=w529, "Rel. hum. (%)"=w528, "a_xyz (g)"=w539, "w_xyz (dps)"=w540, "Status bytes"=w538) -> (w533:T3)
              }
            }
            "chk err" <- w486
            "frm err" <- w487
            n230 = call <vilib>:"Clear Errors.vi"("error in (no error)"=w492, "specific error code to clear (0: all)"=1073676294) -> ("error out"=w491:errorcluster)  [unwired: 4 in, 1 out]
            n231 = local write "Error"(w491) -> ()
            n232 = Greater Or Equal?(x=w482, y=w481) -> (x >= y?=w483:bool)
            n233 = Compound Arithmetic op=OR(w491, "Stop Data", w483) -> (w509:bool)
          }
          n234 = case shown="True" w456 {
            tunnel: [w648 w661] -> w466
            tunnel: w461 -> [w648 w653]
            tunnel: w460 -> [_ w654]
            tunnel: w443 -> [_ w652]
            tunnel: w442 -> [_ w651]
            frame False {
            }
            frame True {
              # "Write any remaining data to disk, then close file"
              n235 = Transpose 2D Array(2D array=w652) -> (transposed array=w658:sgl[][])
              n236 = Build Array (concatenate)(w651, w658) -> (w659:sgl[][])
              n237 = Transpose 2D Array(2D array=w659) -> (transposed array=w660:sgl[][])
              n238 = Array To Spreadsheet String(delimiter (Tab)="\t", array=w660, 3:"%.6f" ("format string")) -> (spreadsheet string=w655:string)
              n239 = Write to Text File(file (use dialog)=w654, text=w655, error in=w653) -> (refnum out=w650:refnum<file>, error out=w649:errorcluster)  [unwired: 1 in, 1 out]
              n240 = Close File(refnum=w650, error in=w649) -> (error out=w661:errorcluster)  [unwired: 1 out]
            }
          }
          n241 = Multiply(x=w446, y=sgl 2000.0) -> (x*y=w447:sgl)
          n242 = To Unsigned Long Integer(number=w447) -> (unsigned 32bit integer=w444:u32)
          n243 = call "24HP_Send Cmd.vi"("Operation"=T2 "d" ("Combo Box"), "Port"=w453) -> ("Error Out"=w450:errorcluster, "Port out"=w451:refnum<visa-resource-name>)  [unwired: 2 in]
          n244 = call "24HP_Clear buffer.vi"("Error in"=w450, "dt for timeout (ms)"=w444, "VISA resource name in"=w451) -> ("Error out"=w448:errorcluster, "VISA resource name out"=w449:refnum<visa-resource-name>)  [unwired: 3 in]
          n245 = call "24HP_Close serial port.vi"("Error in"=w448, "VISA resource name"=w449) -> ("Error out"=w467:errorcluster)  [unwired: 9 in]
        }
      }
      n246 = local write "Stream enabled"(w367) -> ()
      n247 = Merge Errors(w364, w365, w359) -> (w363:errorcluster)
    }
    frame "d" {
      # "Disable USB streaming"
      n248 = flat-sequence {
        tunnel: [w676] -> w669
        tunnel: w668 -> [w676]
        tunnel: w662 -> [w675]
        tunnel: [w670] -> w663
        tunnel: w669 -> [w685]
        tunnel: [w684] -> w667
        tunnel: [TRUE] -> w664
        tunnel: w663 -> [w678]
        frame #0 {
          n249 = Reciprocal(x=w675) -> (1/x=w674:dbl)
          n250 = disable-structure shown="Enabled" {
            frame Disabled {
              n251 = local write "Main"(T4."Data stream" ("Main")) -> ()
            }
            frame Enabled {
            }
          }
          n252 = To Single Precision Float(number=w674) -> (single precision float=w671:sgl)
          n253 = Multiply(x=w671, y=sgl 2000.0) -> (x*y=w672:sgl)
          n254 = To Unsigned Long Integer(number=w672) -> (unsigned 32bit integer=w670:u32)
        }
        frame #1 {
          n255 = local read "COM port"() -> (w686:refnum<visa-resource-name>)
          n256 = call "24HP_Open serial port.vi"("timeout (ms)"=u32 5000, "VISA resource name"=w686) -> ("Error out"=w687:errorcluster, "VISA resource name out"=w688:refnum<visa-resource-name>)  [unwired: 8 in]
          n257 = call "24HP_Send Cmd.vi"("Error In"=w687, "Operation"=w685, "Port"=w688) -> ("Error Out"=w682:errorcluster, "Port out"=w680:refnum<visa-resource-name>)  [unwired: 1 in]
          n258 = call "24HP_Clear buffer.vi"("Error in"=w682, "dt for timeout (ms)"=w678, "VISA resource name in"=w680) -> ("Error out"=w681:errorcluster, "VISA resource name out"=w679:refnum<visa-resource-name>)  [unwired: 3 in]
          n259 = call "24HP_Close serial port.vi"("Error in"=w681, "VISA resource name"=w679) -> ("Error out"=w684:errorcluster)  [unwired: 9 in]
        }
      }
    }
    frame "F" {
      # "Set data rate"
      n260 = flat-sequence {
        tunnel: w698 -> [w701]
        tunnel: [w701] -> w697
        tunnel: w697 -> [w710]
        tunnel: [w707] -> w696
        tunnel: [w709] -> w695
        tunnel: [w751] -> w690
        tunnel: w696 -> [w751]
        tunnel: w695 -> [w749]
        tunnel: [w749] -> w692
        tunnel: [TRUE] -> w691
        frame #0 {
          n261 = local write "Returned data rate (Hz)"(u32 0 ("Returned data rate (Hz)")) -> ()
          n262 = local write "received"(FALSE ("sent")) -> ()
          n263 = local write "Main"(T4."Data rate" ("Main")) -> ()
          n264 = local write "sent"(FALSE ("sent")) -> ()
        }
        frame #1 {
          # "to LE"
          n265 = case shown="14, Default" "Data rate (Hz)" {
            tunnel: [1.0 2.0 4.0 5.0 8.0 10.0 16.0 20.0 25.0 32.0 40.0 50.0 64.0 80.0 100.0 125.0 160.0 200.0 250.0 320.0 400.0 500.0 625.0 800.0 1000.0 1250.0 1600.0 2000.0] -> w707
            frame 0 {
            }
            frame 1 {
            }
            frame 2 {
            }
            frame 3 {
            }
            frame 4 {
            }
            frame 5 {
            }
            frame 6 {
            }
            frame 7 {
            }
            frame 8 {
            }
            frame 9 {
            }
            frame 10 {
            }
            frame 11 {
            }
            frame 12 {
            }
            frame 13 {
            }
            frame 14, Default {
            }
            frame 15 {
            }
            frame 16 {
            }
            frame 17 {
            }
            frame 18 {
            }
            frame 19 {
            }
            frame 20 {
            }
            frame 21 {
            }
            frame 22 {
            }
            frame 23 {
            }
            frame 24 {
            }
            frame 25 {
            }
            frame 26 {
            }
            frame 27 {
            }
          }
          n266 = local read "COM port"() -> (w713:refnum<visa-resource-name>)
          n267 = To Unsigned Long Integer(number=w707) -> (unsigned 32bit integer=w706:u32)
          n268 = Quotient & Remainder(x=u32 1000000, y=w706) -> (floor(x/y)=w705:u32)  [unwired: 1 out]
          n269 = Type Cast(type="", x=w705) -> (*(type *) &x=w719:string)
          n270 = call "24HP_Open serial port.vi"("timeout (ms)"=u32 5000, "VISA resource name"=w713) -> ("Error out"=w714:errorcluster, "VISA resource name out"=w715:refnum<visa-resource-name>)  [unwired: 8 in]
          n271 = Reverse String(1:w719) -> (0:w704:string)
          n272 = call "24HP_Send Cmd + Data.vi"("Error In"=w714, "Data"=w704, "Operation"=w710, "Port"=w715) -> ("Error Out"=w711:errorcluster, "Port out"=w712:refnum<visa-resource-name>)  [unwired: 1 in]
          n273 = call "24HP_Close serial port.vi"("Error in"=w711, "VISA resource name"=w712) -> ("Error out"=w709:errorcluster)  [unwired: 9 in]
        }
        frame #2 {
          n274 = Unbundle By Name(w749) -> ("status"=w750:bool)
          n275 = Not(x=w750) -> (.not. x?=→"sent":bool)
        }
      }
    }
    frame "f" {
      # "Get data rate"
      n276 = flat-sequence {
        tunnel: w761 -> [w764]
        tunnel: [w764] -> w760
        tunnel: w760 -> [w776]
        tunnel: [w779] -> w759
        tunnel: [w781] -> w758
        tunnel: [w788] -> w757
        tunnel: w759 -> [w788]
        tunnel: w758 -> [w786]
        tunnel: [w786] -> w754
        tunnel: [TRUE] -> w753
        frame #0 {
          n277 = local write "received"(FALSE ("sent")) -> ()
          n278 = local write "Main"(T4."Data rate" ("Main")) -> ()
          n279 = local write "sent"(FALSE ("sent")) -> ()
        }
        frame #1 {
          # "to BE"
          n280 = local read "COM port"() -> (w782:refnum<visa-resource-name>)
          n281 = call "24HP_Open serial port.vi"("timeout (ms)"=u32 5000, "VISA resource name"=w782) -> ("Error out"=w777:errorcluster, "VISA resource name out"=w778:refnum<visa-resource-name>)  [unwired: 8 in]
          n282 = call "24HP_Send Cmd.vi"("Error In"=w777, "Operation"=w776, "Port"=w778) -> ("Error Out"=w774:errorcluster, "Port out"=w773:refnum<visa-resource-name>)  [unwired: 1 in]
          n283 = VISA Read(VISA resource name=w773, byte count=u32 4, error in (no error)=w774) -> (VISA resource name out=w771:refnum<visa-resource-name>, read buffer=w766:string, error out=w772:errorcluster)  [unwired: 1 out]
          n284 = call "24HP_Close serial port.vi"("Error in"=w772, "VISA resource name"=w771) -> ("Error out"=w781:errorcluster)  [unwired: 9 in]
          n285 = Reverse String(1:w766) -> (0:w780:string)
          n286 = Type Cast(type=u32 0 ("byte count"), x=w780) -> (*(type *) &x=w768:u32)
          n287 = Quotient & Remainder(x=u32 1000000, y=w768) -> (floor(x/y)=w769:u32)  [unwired: 1 out]
          "Returned data rate (Hz)" <- w769
          n288 = To Double Precision Float(number=w769) -> (double precision float=w779:dbl)
        }
        frame #2 {
          n289 = Unbundle By Name(w786) -> ("status"=w787:bool)
          n290 = Not(x=w787) -> (.not. x?=→"received":bool)
        }
      }
    }
    frame "N" {
      # "Get serial number"
      n291 = flat-sequence {
        tunnel: w792 -> [w798]
        tunnel: [w798] -> w791
        tunnel: [TRUE] -> w795
        tunnel: w791 -> [w804]
        tunnel: [w803] -> w790
        frame #0 {
          n292 = local write "Main"(T4."Action" ("Main")) -> ()
          "Serial number" <- u32 0 ("Numeric")
        }
        frame #1 {
          # "to BE"
          n293 = local read "COM port"() -> (w805:refnum<visa-resource-name>)
          n294 = call "24HP_Open serial port.vi"("timeout (ms)"=u32 5000, "VISA resource name"=w805) -> ("Error out"=w812:errorcluster, "VISA resource name out"=w813:refnum<visa-resource-name>)  [unwired: 8 in]
          n295 = call "24HP_Send Cmd.vi"("Error In"=w812, "Operation"=w804, "Port"=w813) -> ("Error Out"=w810:errorcluster, "Port out"=w811:refnum<visa-resource-name>)  [unwired: 1 in]
          n296 = VISA Read(VISA resource name=w811, byte count=u32 4, error in (no error)=w810) -> (VISA resource name out=w808:refnum<visa-resource-name>, read buffer=w800:string, error out=w807:errorcluster)  [unwired: 1 out]
          n297 = call "24HP_Close serial port.vi"("Error in"=w807, "VISA resource name"=w808) -> ("Error out"=w803:errorcluster)  [unwired: 9 in]
          n298 = Reverse String(1:w800) -> (0:w801:string)
          n299 = Type Cast(type=u32 0 ("byte count"), x=w801) -> (*(type *) &x=w799:u32)
          n300 = local write "Serial number"(w799) -> ()
        }
      }
    }
    frame "R" {
      # "System soft reset"
      n301 = flat-sequence {
        tunnel: w822 -> [w826]
        tunnel: [w826] -> w821
        tunnel: [TRUE] -> w824
        tunnel: w821 -> [w830]
        tunnel: [w829] -> w818
        frame #0 {
          n302 = local write "Main"(T4."Action" ("Main")) -> ()
        }
        frame #1 {
          n303 = local read "COM port"() -> (w831:refnum<visa-resource-name>)
          n304 = call "24HP_Open serial port.vi"("timeout (ms)"=u32 5000, "VISA resource name"=w831) -> ("Error out"=w833:errorcluster, "VISA resource name out"=w834:refnum<visa-resource-name>)  [unwired: 8 in]
          n305 = call "24HP_Send Cmd.vi"("Error In"=w833, "Operation"=w830, "Port"=w834) -> ("Error Out"=w827:errorcluster, "Port out"=w828:refnum<visa-resource-name>)  [unwired: 1 in]
          n306 = call "24HP_Close serial port.vi"("Error in"=w827, "VISA resource name"=w828) -> ("Error out"=w829:errorcluster)  [unwired: 9 in]
        }
      }
      n307 = Enqueue Element(queue=w816, element=T2 "s", error in (no error)=w818) -> (queue out=w815:refnum<queue>, error out=w817:errorcluster)  [unwired: 1 in, 1 out]
    }
    frame "X" {
      # "Exit"
    }
    frame Default {
    }
  }
  "Data out" <- w2
  n308 = Merge Errors(w11, w10, w9) -> (w8:errorcluster)
  n309 = call <vilib>:"Clear Errors.vi"("error in (no error)"=w8, "specific error code to clear (0: all)"=1073676294) -> ("error out"=w3:errorcluster)  [unwired: 4 in, 1 out]
  n310 = local write "Error"(w3) -> ()
  n311 = Release Queue(queue=w4, error in (no error)=w3) -> (error out=→"Error":errorcluster)  [unwired: 1 in, 2 out]
